vi "Darstellende Messwerte erstellen.vi"(1 "file path (use dialog)":path) -> (0 "output array":dbl[][](array[numeric]))   [LabVIEW 2021]
uses:
  <vilib>/Utility/file.llb/Read Delimited Spreadsheet (DBL).vi
  <vilib>/gmath/NI_Gmath.lvlib
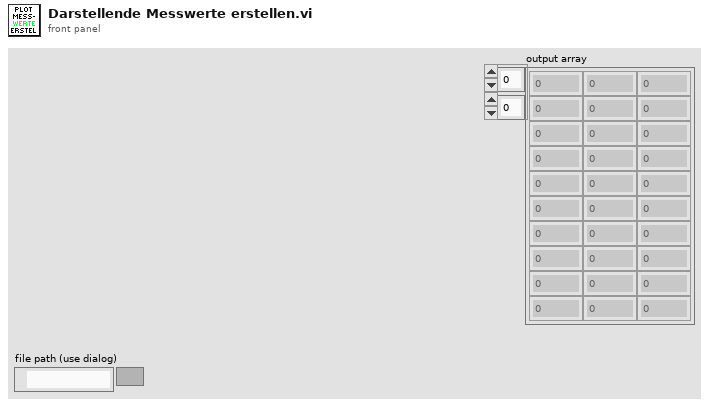
[diagram p1: front panel]
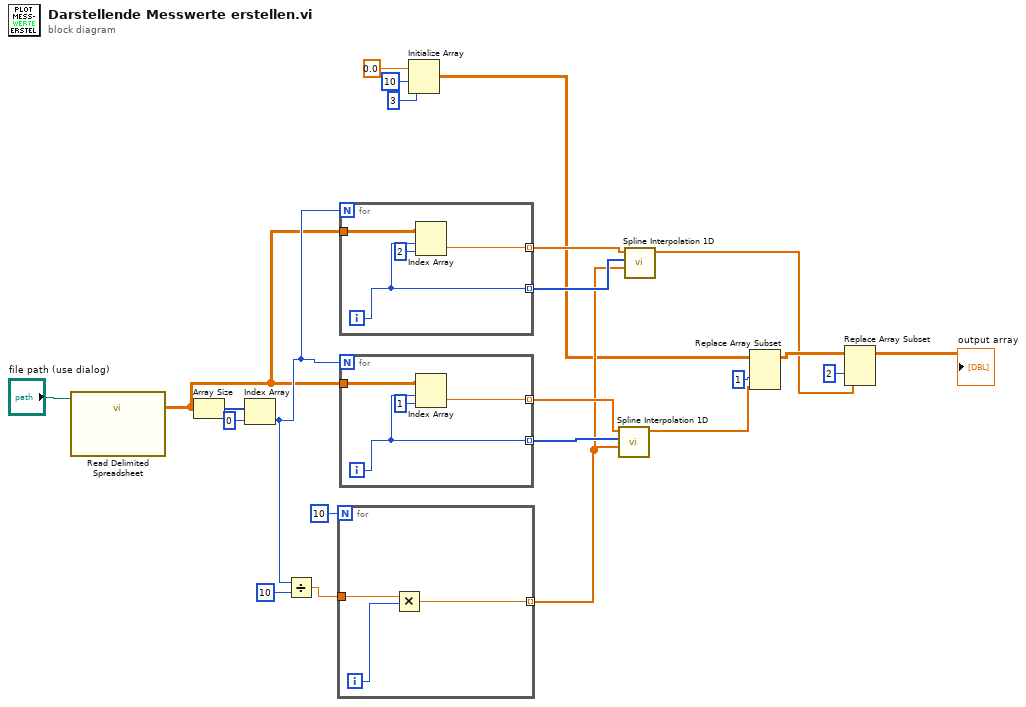
[diagram p0: block diagram]
diagram:
  n1 = call-poly <vilib>:"Read Delimited Spreadsheet.vi"("file path (dialog if empty)"="file path (use dialog)") -> ("all rows"=w11:dbl[][])  [unwired: 9 in, 5 out]
  n2 = Array Size(array=w11) -> (size(s)=w22:i32[])
  n3 = Index Array(array=w22, index=0) -> (element=w12:i32)
  n4 = Divide(x=w12, y=10) -> (x/y=w16:dbl)
  n5 = for {
    N: 10 -> [_]
    tunnel: w16 -> [w26]
    tunnel: [w24] -> w8 mode=indexing
    i -> [w25]
    n6 = Multiply(x=w26, y=w25) -> (x*y=w24:dbl)
  }
  n7 = for {
    N: w12 -> [_]
    tunnel: [w27] -> w9 mode=indexing
    tunnel: w11 -> [w30]
    tunnel: [w28] -> w10 mode=indexing
    i -> [w27]
    n8 = Index Array(array=w30, index (row)=w27, index (col)=2 ("disabled index (col)")) -> (element=w28:dbl)
  }
  n9 = for {
    N: w12 -> [_]
    tunnel: [w31] -> w20 mode=indexing
    tunnel: w11 -> [w34]
    tunnel: [w32] -> w19 mode=indexing
    i -> [w31]
    n10 = Index Array(array=w34, index (row)=w31, index (col)=1 ("disabled index (col)")) -> (element=w32:dbl)
  }
  n11 = Initialize Array(0.0 ("element"), 10 ("dimension size"), 3 ("dimension size")) -> (w7:dbl[][])
  n12 = call <vilib>:"Spline Interpolation 1D.vi"("xi"=w8, "X"=w20, "Y"=w19) -> ("yi"=w5:dbl[])  [unwired: 6 in, 2 out]
  n13 = call <vilib>:"Spline Interpolation 1D.vi"("xi"=w8, "X"=w9, "Y"=w10) -> ("yi"=w2:dbl[])  [unwired: 6 in, 2 out]
  n14 = Replace Array Subset(array=w7, new element=w5, index (col)=1 ("disabled index (col)")) -> (w4:dbl[][])  [unwired: 1 in]
  n15 = Replace Array Subset(array=w4, new element=w2, index (col)=2 ("disabled index (col)")) -> (→"output array":dbl[][])  [unwired: 1 in]
